vi "AFG Report Event.vi"(8 "error in (no error)":errorcluster, 9 "Event Data":variant, 10 "Report Events":T1=enum."Inited", 11 "Unit_Test_AFG in":refnum<class "Unit_Test_AFG.lvclass">) -> (0 "error out":errorcluster, 3 "Unit_Test_AFG out":refnum<class "Unit_Test_AFG.lvclass">)   [LabVIEW 2020, in "Unit_Test_AFG.lvlib" / "Unit_Test_AFG.lvclass"]
uses:
  Unit_Test_AFG.lvclass
  Actor_AFG/AFG_Event.ctl
  Unit_Test_AFG.lvclass/Unit_Test_AFG.ctl
  Actor_AFG/Actor_AFG/Actor_AFG.lvclass
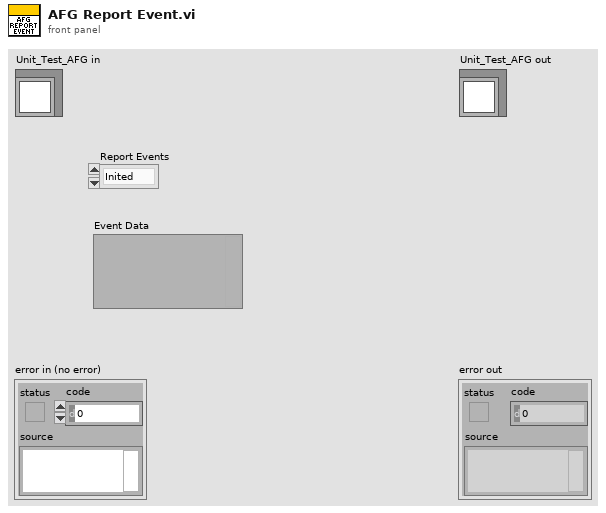
[diagram p1: front panel]
types:
  T1 = typedef "Actor_AFG.lvlib/Actor_AFG.lvclass/AFG_Event.ctl" = enum16{"General Event", "Inited", "Output", "Waveform Set", "DC Configured", "Cycle End", "Error"}
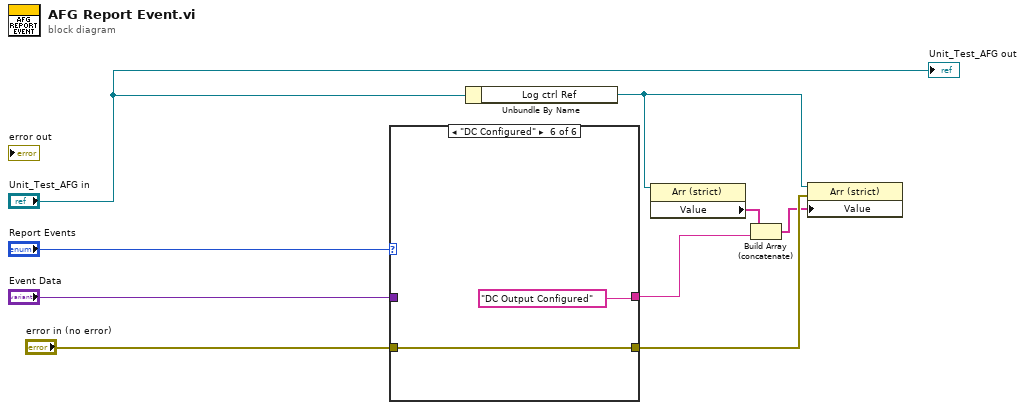
[diagram p0: block diagram]
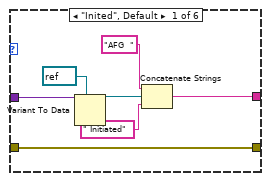
[diagram p2: hidden frame]
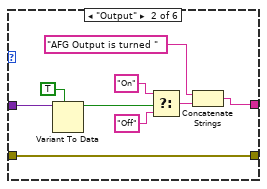
[diagram p3: hidden frame]
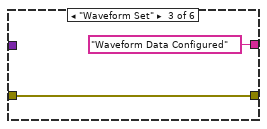
[diagram p4: hidden frame]
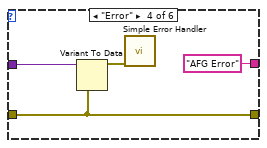
[diagram p5: hidden frame]
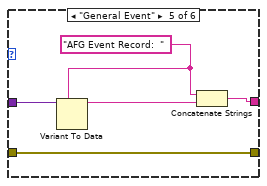
[diagram p6: hidden frame]
diagram:
  n1 = case shown="\"DC Configured\"" "Report Events" {
    tunnel: "Event Data" -> [w16 w24 _ w30 w34 _]
    tunnel: "error in (no error)" -> [w11 w25 w27 w31 w36 w38]
    tunnel: [w11 w25 w27 w31 w36 w38] -> w5
    tunnel: [w10 w17 "Waveform Data Configured" "AFG Error" w32 "DC Output Configured"] -> w3
    frame "Inited", Default {
      n2 = Variant To Data(type=refnum<visa-resource-name> refnum ("VISA resource name"), Variant=w16) -> (data=w14:refnum<visa-resource-name>)  [unwired: 1 in, 1 out]
      n3 = Concatenate Strings("AFG  " ("string"), w14, " Initiated" ("string")) -> (w10:string)
    }
    frame "Output" {
      n4 = Variant To Data(type=TRUE, Variant=w24) -> (data=w22:bool)  [unwired: 1 in, 1 out]
      n5 = Select(t="On", s=w22, f="Off") -> (s? t:f=w19:string)
      n6 = Concatenate Strings("AFG Output is turned ", w19) -> (w17:string)
    }
    frame "Waveform Set" {
    }
    frame "Error" {
      n7 = Variant To Data(type=w31, Variant=w30) -> (data=w29:errorcluster)  [unwired: 1 in, 1 out]
      n8 = call <vilib>:"Simple Error Handler.vi"("error in (no error)"=w29) -> ()  [unwired: 4 in, 5 out]
    }
    frame "General Event" {
      w35 = "AFG Event Record:  "
      n9 = Variant To Data(type=w35, Variant=w34) -> (data=w33:string)  [unwired: 1 in, 1 out]
      n10 = Concatenate Strings(w35, w33) -> (w32:string)
    }
    frame "DC Configured" {
    }
  }
  n11 = Unbundle By Name("Unit_Test_AFG in") -> ("Log ctrl Ref"=w4:refnum<vi>)
  n12 = property class="Arr (strict)"(reference=w4) -> ("Value"=w2:string[])  [unwired: 1 in, 2 out]
  n13 = Build Array (concatenate)(w2, w3) -> (w1:string[])
  n14 = property class="Arr (strict)"(reference=w4, error in=w5, "Value"=w1) -> ()  [unwired: 2 out]
  "Unit_Test_AFG out" <- "Unit_Test_AFG in"
